vi "sub_Sin Acq Point.vi"(5 "Nonlinear Acq.":bool, 7 "Point/Pixel":u16=74, 8 "Effecte Pixel/Line":dbl=512.0, 9 "Fill Fraction":dbl=0.85, 10 "Scanning Speed":dbl=2000.0, 11 "Sample Rate":dbl=120000000.0 format="%#_6p") -> (1 "Total Data Out":u16, 2 "Init Data Out":u16[](array[numeric]), 3 "Init Data Out FXP":fxp<+,18,0>[](array[numeric]) format="%.16g")   [LabVIEW 2015]
panel:
  out "FIX Point/Pixel":fxp<+,18,0>[](array[numeric]) format="%.16g"
  out "Total Pixel/Line":dbl
  out "Average Per Pixel Dis.":dbl[][](graph)
  out "Total Average Per Pixel":dbl[](array[numeric])
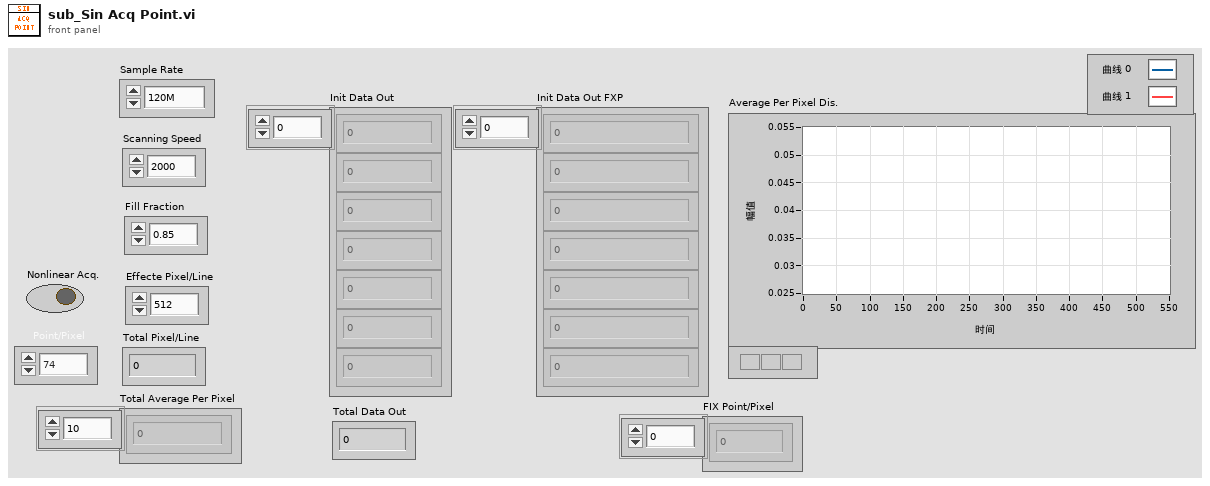
[diagram p1: front panel]
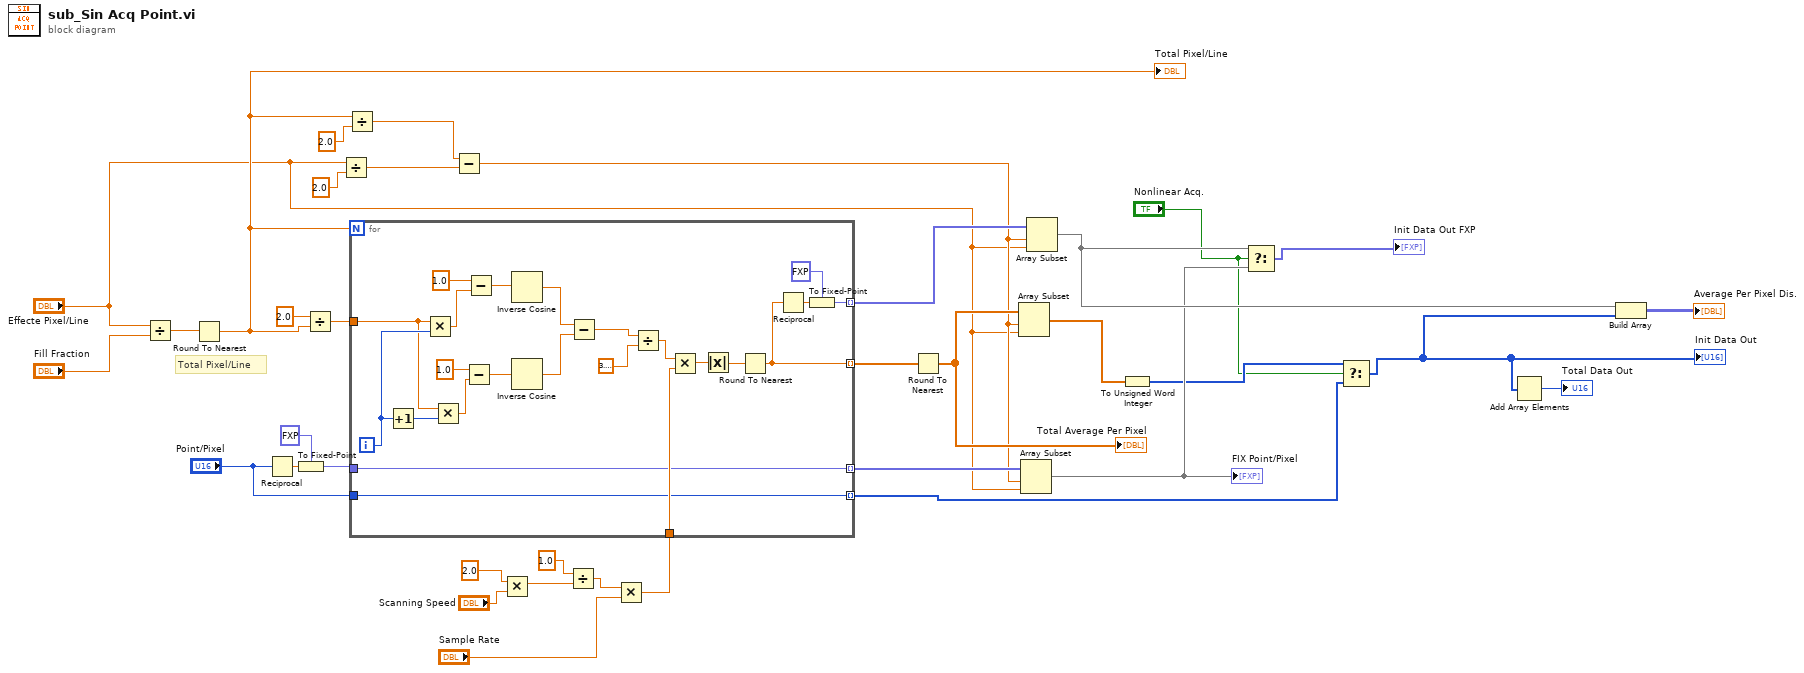
[diagram p0: block diagram]
diagram:
  # "Total Pixel/Line"
  n1 = Divide(x="Effecte Pixel/Line", y="Fill Fraction") -> (x/y=w35:dbl)
  n2 = Round To Nearest(number=w35) -> (nearest integer value=w24:dbl)
  "Total Pixel/Line" <- w24
  n3 = Reciprocal(x="Point/Pixel") -> (1/x=w11:dbl)
  n4 = To Fixed-Point(fixed-point type=fxp<+,18,0> 0.0 ("Y Amplitude"), number=w11) -> (fixed-point=w9:fxp<+,18,0>)
  n5 = Divide(x=2.0, y=w24) -> (x/y=w33:dbl)
  n6 = Divide(x="Effecte Pixel/Line", y=2.0) -> (x/y=w20:dbl)
  n7 = Divide(x=w24, y=2.0) -> (x/y=w22:dbl)
  n8 = Subtract(x=w22, y=w20) -> (x-y=w13:dbl)
  n9 = Multiply(x=2.0, y="Scanning Speed") -> (x*y=w27:dbl)
  n10 = Divide(x=1.0, y=w27) -> (x/y=w26:dbl)
  n11 = Multiply(x=w26, y="Sample Rate") -> (x*y=w31:dbl)
  n12 = for {
    N: w24 -> [_]
    tunnel: w33 -> [w50]
    tunnel: w31 -> [w45]
    tunnel: [w39] -> w29 mode=indexing
    tunnel: [w42] -> w16 mode=indexing
    tunnel: [w38] -> w14 mode=indexing
    tunnel: w9 -> [w38]
    tunnel: [w37] -> w4 mode=indexing
    tunnel: "Point/Pixel" -> [w37]
    i -> [w53]
    n13 = Increment(x=w53) -> (x+1=w52:i32)
    n14 = Multiply(x=w50, y=w53) -> (x*y=w55:dbl)
    n15 = Multiply(x=w50, y=w52) -> (x*y=w51:dbl)
    n16 = Subtract(x=1.0, y=w51) -> (x-y=w49:dbl)
    n17 = Subtract(x=1.0, y=w55) -> (x-y=w56:dbl)
    n18 = Inverse Cosine(1:w56) -> (0:w59:dbl)
    n19 = Inverse Cosine(1:w49) -> (0:w58:dbl)
    n20 = Subtract(x=w59, y=w58) -> (x-y=w48:dbl)
    n21 = Divide(x=w48, y=3.141592653589793) -> (x/y=w46:dbl)
    n22 = Multiply(x=w46, y=w45) -> (x*y=w41:dbl)
    n23 = Absolute Value(x=w41) -> (abs(x)=w40:dbl)
    n24 = Round To Nearest(number=w40) -> (nearest integer value=w39:dbl)
    n25 = Reciprocal(x=w39) -> (1/x=w44:dbl)
    n26 = To Fixed-Point(fixed-point type=fxp<+,18,0> 0.0 ("Y Amplitude"), number=w44) -> (fixed-point=w42:fxp<+,18,0>)
  }
  n27 = Round To Nearest(number=w29) -> (nearest integer value=w17:dbl[])
  "Total Average Per Pixel" <- w17
  n28 = Array Subset(array=w17, index=w13, length="Effecte Pixel/Line") -> (w18:dbl[])
  n29 = Array Subset(array=w14, index=w13, length="Effecte Pixel/Line") -> (w7:fxp<+,18,0>[])
  "FIX Point/Pixel" <- w7
  n30 = Array Subset(array=w16, index=w13, length="Effecte Pixel/Line") -> (w8:fxp<+,18,0>[])
  n31 = To Unsigned Word Integer(number=w18) -> (unsigned 16bit integer=w2:u16[])
  n32 = Select(t=w8, s="Nonlinear Acq.", f=w7) -> (s? t:f=→"Init Data Out FXP":fxp<+,18,0>[])
  n33 = Select(t=w2, s="Nonlinear Acq.", f=w4) -> (s? t:f=w5:u16[])
  "Init Data Out" <- w5
  n34 = Add Array Elements(numeric array=w5) -> (sum=→"Total Data Out":u16)
  n35 = Build Array(w8, w5) -> (→"Average Per Pixel Dis.":fxp<+,34,16>[][])
